vi "Finish.vi"   [LabVIEW 2013]
doc: "This VI is called just before exiting. It is expected to close I/O refnum, save collected data, etc."
uses:
  <vilib>/Rock Robotics/WPI/Joystick/WPI_JoystickGetSetRefNum.vi
types:
  T1 = typedef "WPI_JoystickDevRef.ctl" = cluster{"Device":T2}
  T2 = typedef "WPI_JoystickDeviceEnum.ctl" = enum16{"USB 1", "USB 2", "USB 3", "USB 4", "Kinect 1", "Kinect 2"}
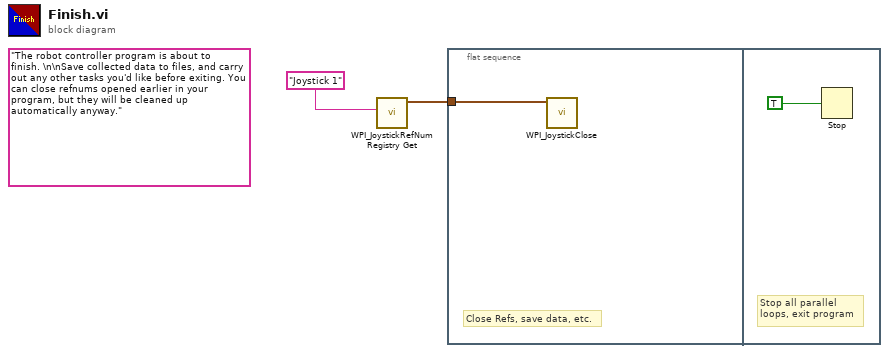
[diagram p0: block diagram]
diagram:
  (unwired) "The robot controller program is about to finish. \n\nSave collected data to files, and carry out any other tasks you'd like before exiting. You can close refnums opened earlier in your program, but they will be cleaned up automatically anyway."
  n1 = call <vilib>:"WPI_JoystickRefNum Registry Get.vi"("refnum name"="Joystick 1") -> ("JoystickDevRef"=w1:T1)  [unwired: 1 in, 9 out]
  n2 = flat-sequence {
    tunnel: w1 -> [w3]
    frame #0 {
      # "Close Refs, save data, etc."
      n3 = call <vilib>:"WPI_JoystickClose.vi"("JoystickDevRef"=w3) -> ()  [unwired: 11 out]
    }
    frame #1 {
      # "Stop all parallel\nloops, exit program"
      n4 = Stop(stop? (T)=TRUE ("Quit")) -> ()
    }
  }
